vi "Parse Request-JSONtext.vi"(8 "error in (no error)":errorcluster, 10 "<JSON> Request":string) -> (0 "error out":errorcluster, 1 "params":string, 2 "method":string, 4 "id":string)   [LabVIEW 2019, in "JSON-RPC.lvclass"]
uses:
  JSON-RPC.lvclass
  66b5d778-a0b8-403e-b727-bb36a32d382a.vi
  6814ee06-2257-4c2f-8f04-31d91309bef7.vi
  f1c5ac56-d3e8-467f-aff4-e25fa4ac2541.vi
  <vilib>/JDP Science/JSONtext/JSON text to Variant.vi
  <vilib>/JDP Science/JSONtext/LVClass Serializer/JSONtext LVClass Serializer.lvclass
  <vilib>/JDP Science/JSONtext/JSONtext.lvlib
  523bbeac-5bfa-4355-a479-ec0e355c2dae.vi
  5dfc14ef-dff6-4e36-b5f1-09fb62becacc.vi
  f339b867-7010-45a6-b71e-b2a9da4366e1.vi
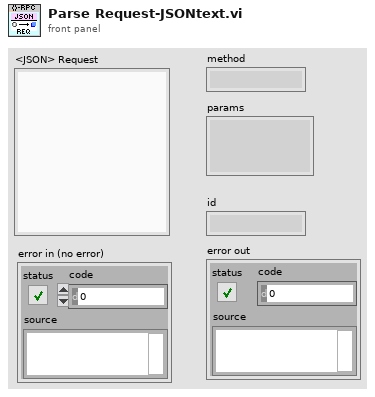
[diagram p1: front panel]
types:
  T1 = cluster{"jsconrpc":string, "method":string, "params":string, "id":string}
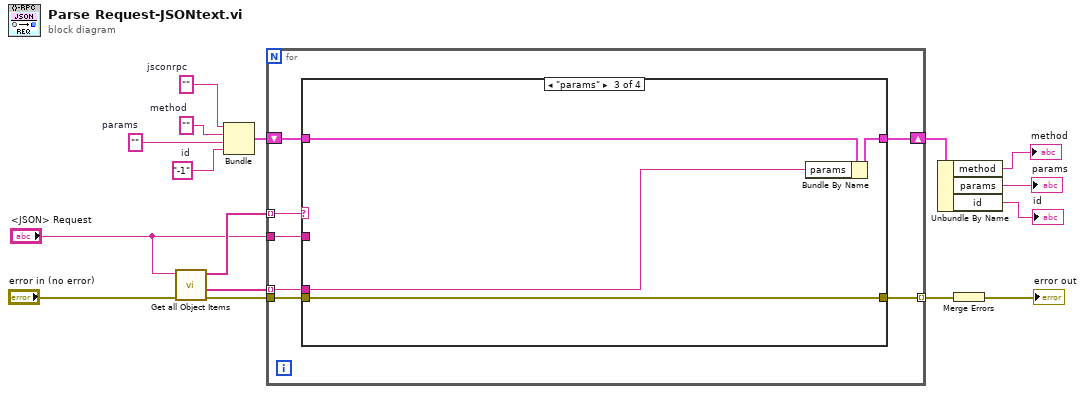
[diagram p0: block diagram]
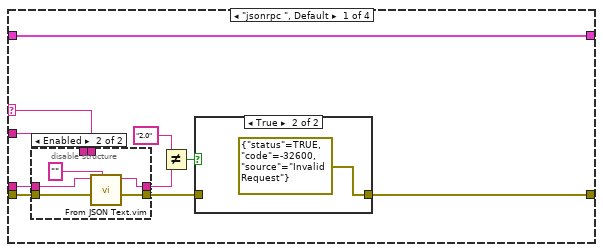
[diagram p2: hidden frame]
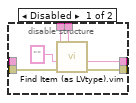
[diagram p3: hidden frame]
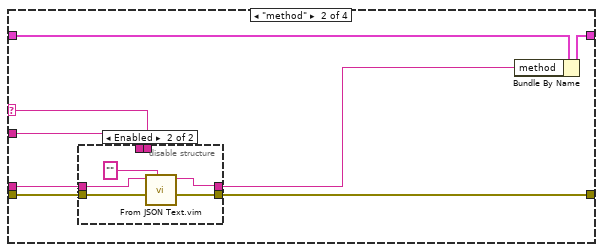
[diagram p5: hidden frame]
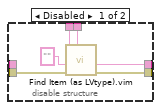
[diagram p6: hidden frame]
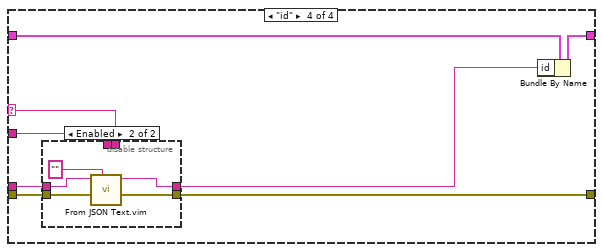
[diagram p7: hidden frame]
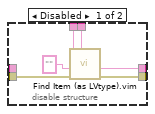
[diagram p8: hidden frame]
diagram:
  w14 = "-1"  # id
  w13 = ""  # params
  w12 = ""  # jsconrpc
  w11 = ""  # method
  n1 = call <vilib>:"Get all Object Items.vi"("error in (no error)"="error in (no error)", "JSON"="<JSON> Request") -> ("error out"=w8:errorcluster, "<JSON>"=w3:string[], "Item Names"=w10:string[])  [unwired: 6 in, 1 out]
  n2 = Bundle("jsconrpc"=w12, "method"=w11, "params"=w13, "id"=w14) -> (w15:T1)  [unwired: 1 in]
  n3 = for {
    tunnel: w3 -> [w22] mode=indexing
    tunnel: w10 -> [w23] mode=indexing
    tunnel: w8 -> [w21]
    tunnel: [w20] -> w9 mode=indexing
    tunnel: "<JSON> Request" -> [w19]
    shift-right: [w17] -> w16
    shift-left: w15 -> [w18]
    n4 = case shown="\"params\"" w23 {
      selector: w23 -> [w28 w53 _ w77]
      tunnel: w22 -> [w24 w47 w66 w70]
      tunnel: w21 -> [w30 w54 w67 w76]
      tunnel: [w31 w52 w67 w75] -> w20
      tunnel: w19 -> [w25 w48 _ w72]
      tunnel: w18 -> [w26 w51 w69 w74]
      tunnel: [w26 w50 w68 w73] -> w17
      frame "jsonrpc ", Default {
        n5 = disable-structure shown="Enabled" {
          disable-tunnel: w30 -> [w39 w40]
          disable-tunnel: [w38 w41] -> w29
          disable-tunnel: w28 -> [w37 _]
          disable-tunnel: [w36 w42] -> w27
          disable-tunnel: w25 -> [w34 _]
          disable-tunnel: w24 -> [_ w43]
          frame Disabled {
            n6 = call "Find Item (as LVtype).vim"("$Path or Item Name"=w37, "error in (no error)"=w39, "Data Type and Default Value"="" ("x"), "JSON"=w34) -> ("error out"=w38:errorcluster, "Data"=w36:string)  [unwired: 4 in, 2 out]
          }
          frame Enabled {
            n7 = call "From JSON Text.vim"("Data Type and Default Value"="", "error in (no error)"=w40, "JSON"=w43) -> ("error out"=w41:errorcluster, "Data out"=w42:string)  [unwired: 7 in]
          }
        }
        n8 = Not Equal?(x="2.0", y=w27) -> (x != y?=w32:bool)
        n9 = case shown="True" w32 {
          tunnel: w29 -> [w45 _]
          tunnel: [w45 errorcluster {"status"=TRUE, "code"=-32600, "source"="Invalid Request"} ("error out")] -> w31
          frame False {
          }
          frame True {
          }
        }
      }
      frame "method" {
        n10 = disable-structure shown="Enabled" {
          disable-tunnel: w54 -> [w60 w64]
          disable-tunnel: w53 -> [w58 _]
          disable-tunnel: [w57 w61] -> w52
          disable-tunnel: [w56 w62] -> w49
          disable-tunnel: w48 -> [w55 _]
          disable-tunnel: w47 -> [_ w63]
          frame Disabled {
            n11 = call "Find Item (as LVtype).vim"("$Path or Item Name"=w58, "error in (no error)"=w60, "Data Type and Default Value"="" ("x"), "JSON"=w55) -> ("error out"=w57:errorcluster, "Data"=w56:string)  [unwired: 4 in, 2 out]
          }
          frame Enabled {
            n12 = call "From JSON Text.vim"("Data Type and Default Value"="", "error in (no error)"=w64, "JSON"=w63) -> ("error out"=w61:errorcluster, "Data out"=w62:string)  [unwired: 7 in]
          }
        }
        n13 = Bundle By Name(cluster=w51, "method"=w49) -> (w50:T1)
      }
      frame "params" {
        n14 = Bundle By Name(cluster=w69, "params"=w66) -> (w68:T1)
      }
      frame "id" {
        n15 = disable-structure shown="Enabled" {
          disable-tunnel: w77 -> [w83 _]
          disable-tunnel: w76 -> [w82 w87]
          disable-tunnel: [w81 w85] -> w75
          disable-tunnel: w72 -> [w79 _]
          disable-tunnel: [w78 w86] -> w71
          disable-tunnel: w70 -> [_ w88]
          frame Disabled {
            n16 = call "Find Item (as LVtype).vim"("$Path or Item Name"=w83, "error in (no error)"=w82, "Data Type and Default Value"="", "JSON"=w79) -> ("error out"=w81:errorcluster, "Data"=w78:string)  [unwired: 4 in, 2 out]
          }
          frame Enabled {
            n17 = call "From JSON Text.vim"("Data Type and Default Value"="", "error in (no error)"=w87, "JSON"=w88) -> ("error out"=w85:errorcluster, "Data out"=w86:string)  [unwired: 7 in]
          }
        }
        n18 = Bundle By Name(cluster=w74, "id"=w71) -> (w73:T1)
      }
    }
  }
  n19 = Unbundle By Name(w16) -> ("method"=→"method":string, "params"=→"params":string, "id"=→"id":string)
  n20 = Merge Errors(w9) -> (→"error out":errorcluster)
